vi "Actor Core.vi"(8 "error in":errorcluster, 11 "SCADA Communications in":refnum<class "SCADA Communications.lvclass">) -> (0 "error out":errorcluster, 3 "Actor out":refnum<class "Actor.lvclass">)   [LabVIEW 2015, in "SCADA Communcations Actor.lvlib" / "SCADA Communications.lvclass"]
doc: "(<B>Filename</B>: Actor Framework.lvlib:Actor.lvclass:Actor Core.vi)\n\nReceives messages to the actor, reacts to them, and initiates any error handling that may shut the actor down.\n\nDescendant classes may override this VI to append parallel tasks for the actor to complete while it handles messages. Overrides use the Call Parent Method node."
uses:
  SCADA Communications.lvclass
  <vilib>/ActorFramework/Actor/Actor.lvclass
  SCADA Communications.lvclass/SCADA Communications.ctl
  TCPIP Communications Framework/TCPIP Communications/TCPIP Communications.lvclass
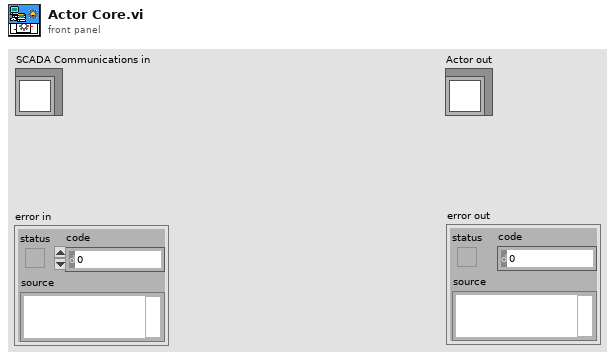
[diagram p1: front panel]
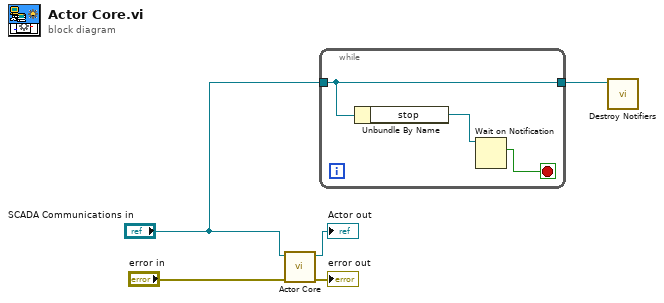
[diagram p0: block diagram]
diagram:
  n1 = call-parent "Actor Core.vi"("error in"="error in", "TCPIP Communications in"="SCADA Communications in") -> ("error out"=→"error out":errorcluster, "Actor out"=→"Actor out":refnum<class "Actor.lvclass">)  [unwired: 8 in]
  n2 = while {
    tunnel: "SCADA Communications in" -> [w8]
    tunnel: [w8] -> w1
    stop <- w6 stop-if-true
    n3 = Unbundle By Name(w8) -> ("stop"=w7:refnum<notifier>)
    n4 = Wait on Notification(notifier=w7) -> (notification=w6:bool)  [unwired: 3 in, 3 out]
  }
  n5 = call "Destroy Notifiers.vi"("SCADA Communications in"=w1) -> ()  [unwired: 10 in, 1 out]
